vi "Global grandezze linea.vi"() -> ()   [LabVIEW 2019]
uses:
  TypeDef/Grandezze banco.ctl
panel:
  out "Grandezze 2":T1
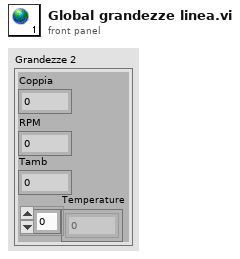
[diagram p1: front panel]
types:
  T1 = typedef "Grandezze banco.ctl" = cluster{"Coppia":dbl, "RPM":dbl, "Tamb":dbl, "Temperature":dbl[]}
diagram:
